vi "Data trimming.vi"(7 "start pixel":i32, 8 "error in":errorcluster, 9 "#pixels to save":i32=300, 10 "#A-lines":i32=2048, 11 "2D Array in":sgl[][](array[numeric])) -> (0 "error out":errorcluster, 2 "time":dbl, 3 "array for saving":sgl[](array[numeric]))   [LabVIEW 2018]
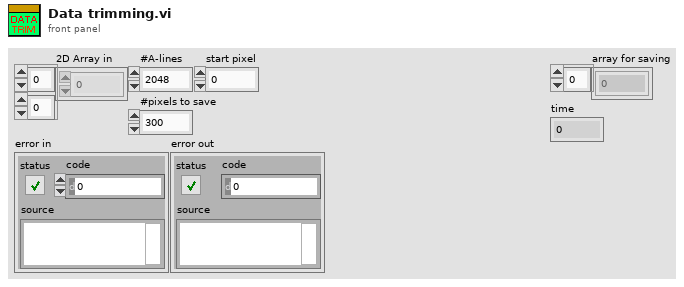
[diagram p1: front panel]
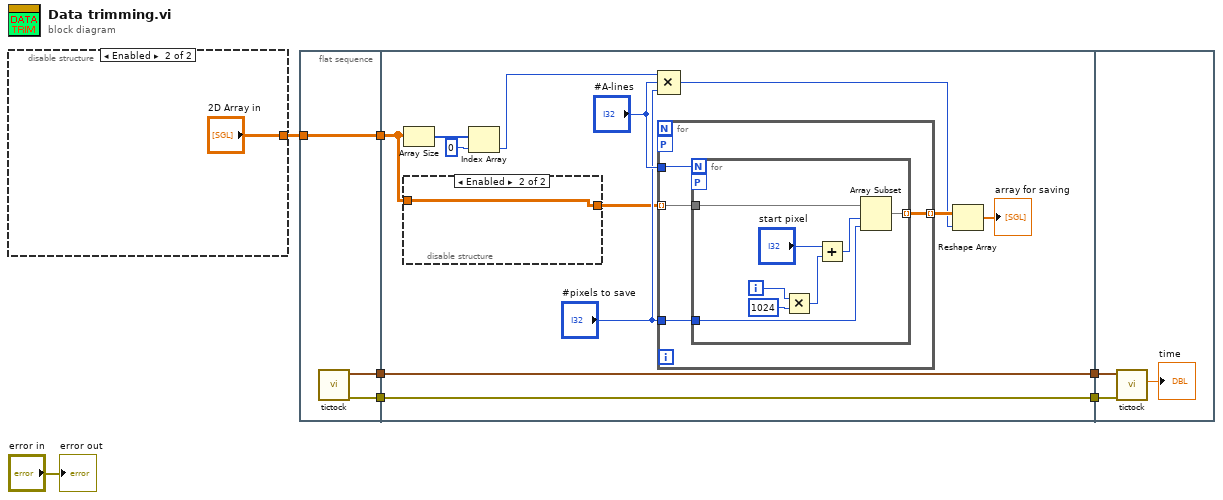
[diagram p0: block diagram]
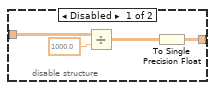
[diagram p2: hidden frame]
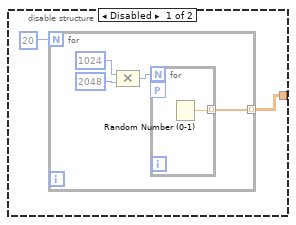
[diagram p3: hidden frame]
diagram:
  n1 = disable-structure shown="Enabled" {
    disable-tunnel: [w8 "2D Array in"] -> w6
    frame Disabled {
      n2 = for {
        N: 20 -> [_]
        tunnel: [w10] -> w8 mode=indexing
        n3 = Compound Arithmetic op=MULTIPLY(1024, 2048) -> (w11:i32)
        n4 = for {
          N: w11 -> [_]
          tunnel: [w14] -> w10 mode=indexing
          workers-P: _ -> [_]
          n5 = Random Number (0-1)() -> (number: 0 to 1=w14:dbl)
        }
      }
    }
    frame Enabled {
    }
  }
  n6 = flat-sequence {
    tunnel: w6 -> [w18]
    tunnel: [w18] -> w5
    tunnel: [w17] -> w4
    tunnel: [w16] -> w3
    tunnel: w5 -> [w20]
    tunnel: [w25] -> w2
    tunnel: w4 -> [w25]
    tunnel: [w21] -> w1
    tunnel: w3 -> [w21]
    tunnel: w2 -> [w50]
    tunnel: w1 -> [w49]
    frame #0 {
      n7 = call "tictock.vi"() -> ("error out"=w16:errorcluster, "seconds since 1Jan1904"=w17:timestamp)  [unwired: 9 in, 1 out]
    }
    frame #1 {
      n8 = Array Size(array=w20) -> (size(s)=w28:i32[])
      n9 = disable-structure shown="Enabled" {
        disable-tunnel: w20 -> [w34 w35]
        disable-tunnel: [w31 w35] -> w19
        frame Disabled {
          n10 = Divide(x=w34, y=sgl 1000.0) -> (x/y=w32:sgl[][])
          n11 = To Single Precision Float(number=w32) -> (single precision float=w31:sgl[][])
        }
        frame Enabled {
        }
      }
      n12 = Index Array(array=w28, index=0) -> (element=w26:i32)
      n13 = Compound Arithmetic op=MULTIPLY(w26, "#A-lines", "#pixels to save") -> (w23:i32)
      n14 = for {
        tunnel: w19 -> [w39] mode=indexing
        workers-P: _ -> [_]
        tunnel: [w38] -> w24 mode=indexing
        tunnel: "#A-lines" -> [w37]
        tunnel: "#pixels to save" -> [w36]
        n15 = for {
          N: w37 -> [_]
          tunnel: w39 -> [w45]
          workers-P: _ -> [_]
          tunnel: [w44] -> w38 mode=indexing
          tunnel: w36 -> [w43]
          i -> [w47]
          n16 = Multiply(x=w47, y=1024) -> (x*y=w41:i32)
          n17 = Add(x="start pixel", y=w41) -> (x+y=w40:i32)
          n18 = Array Subset(array=w45, index=w40, length=w43) -> (w44:sgl[])
        }
      }
      n19 = Reshape Array(w24, w23) -> (→"array for saving":sgl[])
    }
    frame #2 {
      n20 = call "tictock.vi"("error in (no error)"=w49, "seconds since 1Jan1904 2"=w50) -> ("Numeric"=→"time":dbl)  [unwired: 7 in, 2 out]
    }
  }
  "error out" <- "error in"
